vi "ExFileReadNConvertToU16.vi"() -> ()   [LabVIEW 2010]
panel:
  in  "Full File Name":path=path "C:/Program Files/SIToolKit/LabVIEW/Data Files/Color.SPE"
  in  "?":bool
  in  "FileType":u32=67371008
  out "error out":errorcluster
  in  "error in (no error)":errorcluster
  # "ExReadFileNconvertToU16.vi\nThis example will read in a file of the\nselected data type and display as u16 frame.\nWhen finished viewing data, make sure to\nuse the STOP button to close the display."
  # "File Types:\nSPE = 67371008\nTIF   = 67174400\nPMI  = 67436544"
  # "Browse match pattern is set to *.tif.  Modify this if different file type is needed."
  # "This will properly close\nthe image and\ndeallocate memory."
  # "NOTICE\n\nTHIS VI REQUIRES THAT THE TOOLKIT\nBE UNLOADED BY RUNNING THE\n VI EXCLOSEGLOBALCAM.VI\n BEFORE LEAVING LABVIEW."
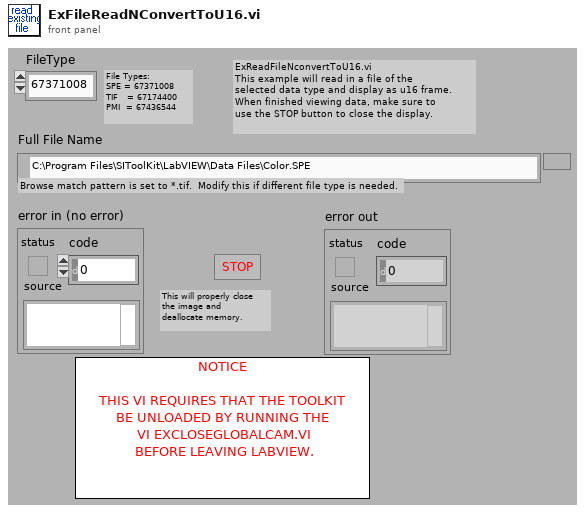
[diagram p1: front panel]
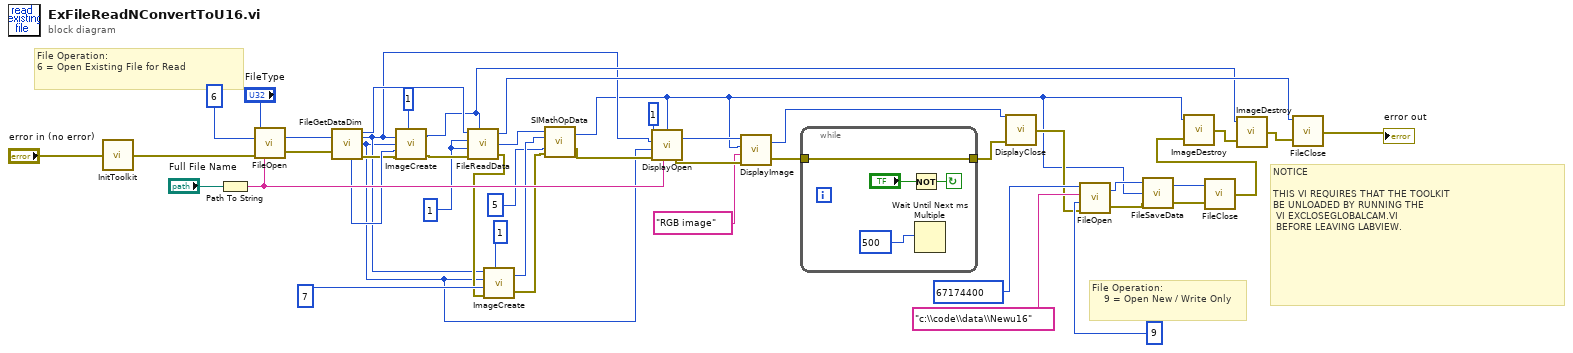
[diagram p0: block diagram]
diagram:
  w34 = 1
  # "NOTICE\n\nTHIS VI REQUIRES THAT THE TOOLKIT\nBE UNLOADED BY RUNNING THE\n VI EXCLOSEGLOBALCAM.VI\n BEFORE LEAVING LABVIEW."
  # "File Operation:\n    9 = Open New / Write Only"
  # "File Operation:\n6 = Open Existing File for Read"
  n1 = call <userlib>:"InitToolkit.vi"("error in"="error in (no error)") -> ("error out"=w44:errorcluster)
  n2 = Path To String(path="Full File Name") -> (string=w37:string)
  n3 = call <userlib>:"FileOpen.vi"("error in"=w44, "File Operations"=u32 6 ("File Operation"), "FileName"=w37, "File Type"="FileType") -> ("error out"=w42:errorcluster, "File Handle"=w41:u32)
  n4 = call <userlib>:"FileGetDataDim.vi"("File Handle"=w41, "error in"=w42) -> ("Data Type"=w24:u32, "File Handle"=w36:u32, "X dim"=w4:u32, "Y dim"=w3:u32, "error out"=w20:errorcluster)  [unwired: 1 out]
  n5 = call <userlib>:"ImageCreate.vi"("X dimension"=w4, "Y dimension"=w3, "Data Type"=w24, "error in"=w20, "Number Of Frames"=1) -> ("Image Handle"=w26:u32, "error out"=w35:errorcluster)
  n6 = call <userlib>:"FileReadData.vi"("File Handle"=w36, "Start Frame"=w34, "End Frame"=w34, "error in"=w35, "Image Handle"=w26) -> ("File Handle"=w33:u32, "Image Handle"=w17:u32, "error out"=w21:errorcluster)
  n7 = call <userlib>:"ImageCreate.vi"("X dimension"=w4, "Y dimension"=w3, "Data Type"=7, "error in"=w21, "Number Of Frames"=1) -> ("Image Handle"=w18:u32, "error out"=w19:errorcluster)
  n8 = call <userlib>:"SIMathOpData.vi"("error in (no error)"=w19, "Operation"=5, "Result Handle"=w18, "Data Handle"=w17) -> ("error out"=w15:errorcluster, "Result Handle"=w2:u32)
  n9 = call <userlib>:"DisplayOpen.vi"("Display Title"=w37, "Image Handle"=w2, "error in"=w15, "Display Height"=w3, "Display Width"=w4, "Display Type"=1) -> ("error out"=w32:errorcluster, "Display Handle"=w31:u32)
  n10 = call <userlib>:"DisplayImage.vi"("error in"=w32, "Title"="RGB image", "Image Handle"=w2, "Display Handle"=w31) -> ("error out"=w25:errorcluster, "Display Handle"=w30:u32)
  n11 = while {
    tunnel: w25 -> [w47]
    tunnel: [w47] -> w7
    stop <- w49 continue-if-true
    n12 = Not(x="?") -> (.not. x?=w49:bool)
    n13 = Wait Until Next ms Multiple(millisecond multiple=500) -> ()  [unwired: 1 out]
  }
  n14 = call <userlib>:"DisplayClose.vi"("error in"=w7, "Display Handle"=w30) -> ("error out"=w6:errorcluster)
  n15 = call <userlib>:"FileOpen.vi"("error in"=w6, "File Operations"=9, "FileName"="c:\\code\\data\\Newu16", "File Type"=67174400) -> ("error out"=w14:errorcluster, "File Handle"=w12:u32)
  n16 = call <userlib>:"FileSaveData.vi"("error in"=w14, "Image Handle"=w2, "File Handle"=w12) -> ("error out"=w13:errorcluster, "File Handle"=w11:u32)
  n17 = call <userlib>:"FileClose.vi"("error in"=w13, "File Handle"=w11) -> ("error out"=w5:errorcluster)
  n18 = call <userlib>:"ImageDestroy.vi"("error in"=w5, "Data handle"=w2) -> ("error out"=w29:errorcluster)
  n19 = call <userlib>:"ImageDestroy.vi"("error in"=w29, "Data handle"=w26) -> ("error out"=w28:errorcluster)
  n20 = call <userlib>:"FileClose.vi"("error in"=w28, "File Handle"=w33) -> ("error out"=→"error out":errorcluster)
